vi "Enqueue.vi"() -> ()   [LabVIEW 2013]
panel:
  out "Data":variant
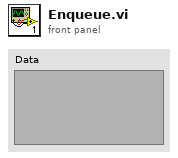
[diagram p1: front panel]
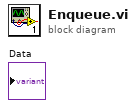
[diagram p0: block diagram]
diagram:
